vi "Pointer.New.vi"(8 "error in (no error)":errorcluster, 11 "size in bytes":u64) -> (0 "error out":errorcluster, 3 "pointer":u64 format="%016x")   [LabVIEW 2016, in "VeriStand Data.lvlib"]
doc: "Obtains a new pointer from the LabVIEW Memory Manager."
uses:
  VeriStand Data.lvlib
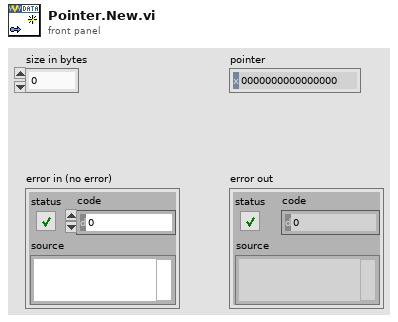
[diagram p1: front panel]
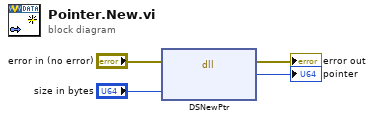
[diagram p0: block diagram]
diagram:
  n1 = dll-call lib="LabVIEW" fn="DSNewPtr"(error in="error in (no error)", "size"="size in bytes") -> (error out=→"error out":errorcluster, "ptr"=→"pointer":u64)  [unwired: 3 in, 1 out]
